vi "Array Size.vi"() -> ()   [LabVIEW 2016]
panel:
  out "Array Size":dbl
  in  "Array":dbl[](array[numeric])
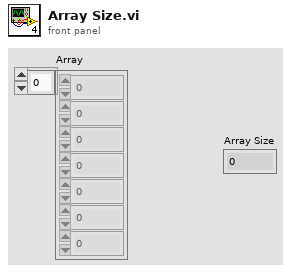
[diagram p1: front panel]
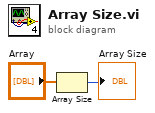
[diagram p0: block diagram]
diagram:
  n1 = Array Size(array="Array") -> (size(s)=→"Array Size":i32)
